vi "GenerateDefaultChannelList.vi"(11 "Channels per Dynamic Module":i32[](array[numeric])) -> (3 "default channel list":string[](array[string]))   [LabVIEW 2017, in "CmsAcquisition.lvlib"]
uses:
  <vilib>/addons/InsightCM/Devices/Shared/Cms/CmsAcquisition/CmsAcquisition.lvlib
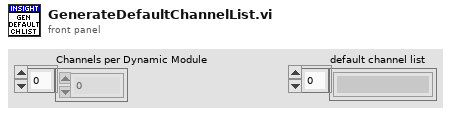
[diagram p1: front panel]
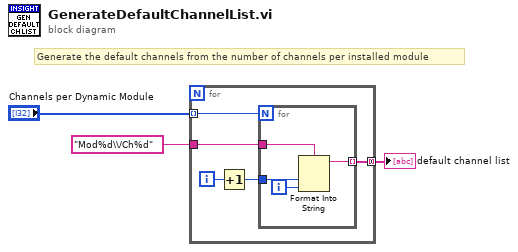
[diagram p0: block diagram]
diagram:
  # "Generate the default channels from the number of channels per installed module"
  n1 = for {
    tunnel: "Mod%d\\/Ch%d" -> [w8]
    tunnel: [w5] -> w2 mode=concatenating
    tunnel: "Channels per Dynamic Module" -> [w4] mode=indexing
    i -> [w7]
    n2 = Increment(x=w7) -> (x+1=w6:i32)
    n3 = for {
      N: w4 -> [_]
      tunnel: w8 -> [w12]
      tunnel: w6 -> [w10]
      tunnel: [w9] -> w5 mode=indexing
      i -> [w11]
      n4 = Format Into String(format string=w12, w10, w11) -> (resulting string=w9:string)  [unwired: 2 in, 1 out]
    }
  }
  "default channel list" <- w2
